vi "WFT Get Version.vi"(8 "Error In":errorcluster) -> (0 "Error Out":errorcluster, 1 "szVersion":string, 2 "ret":i32)   [LabVIEW 2020, in "lv_waveforms_toolkit.lvlib"]
uses:
  lv_waveforms_toolkit.lvlib
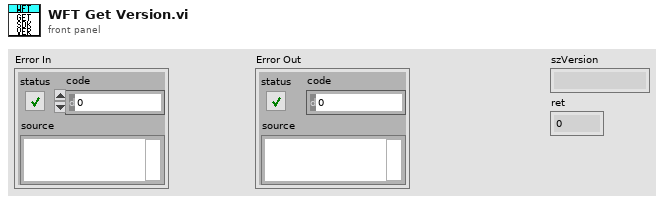
[diagram p1: front panel]
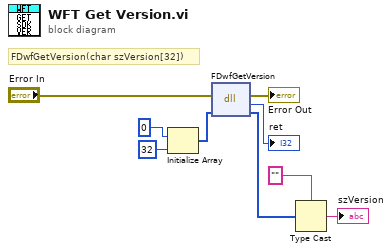
[diagram p0: block diagram]
diagram:
  # "FDwfGetVersion(char szVersion[32])"
  n1 = Initialize Array(u8 0, 32 ("dimension size")) -> (w7:u8[])
  n2 = dll-call lib="dwf" fn="FDwfGetVersion"(error in="Error In", "szVersion"=w7) -> (error out=→"Error Out":errorcluster, "return type"=→"ret":i32, "szVersion"=w6:u8[])  [unwired: 2 in, 1 out]
  n3 = Type Cast(type="", x=w6) -> (*(type *) &x=→"szVersion":string)
